vi "datastringtoformat.vi"(0 "object in":refnum<class "interface.lvclass">, 1 "data[0]":string, 5 "error in (no error)":errorcluster) -> (14 "object out":refnum<class "interface.lvclass">, 15 "time stamp":timestamp format="%<%Y/%m/%d %H:%M:%S>T", 19 "error out":errorcluster)   [LabVIEW 2016, in "interface.lvclass"]
uses:
  interface.lvclass
  <vilib>/Utility/miscctls.llb/LVDateTimeRec.ctl
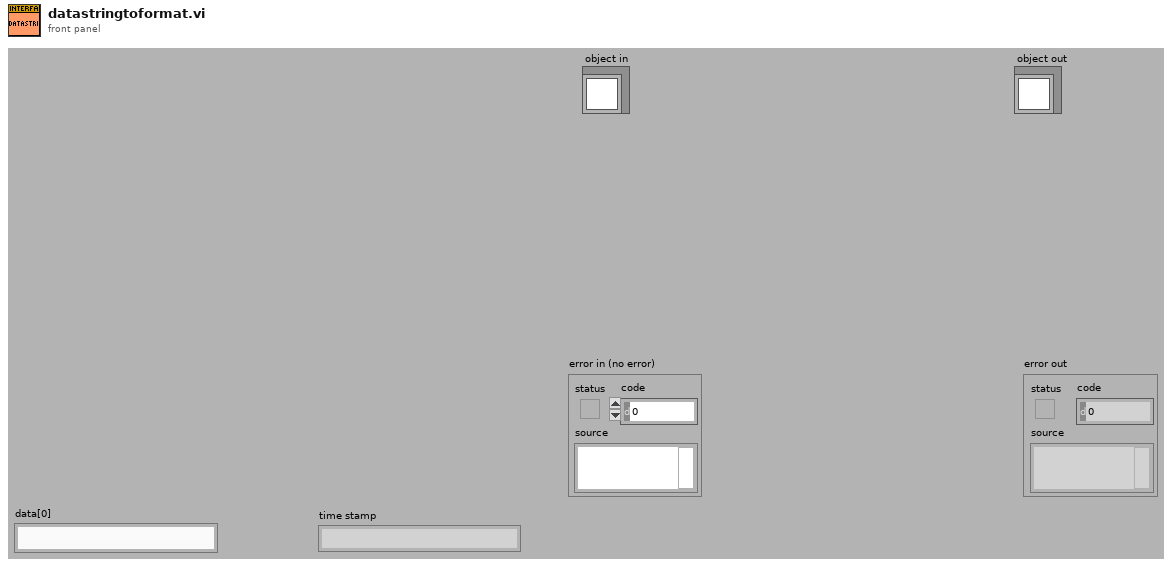
[diagram p1: front panel]
types:
  T1 = typedef "LVDateTimeRec.ctl" = cluster{"fractional second":dbl, "second":i32, "minute":i32, "hour":i32, "day of month":i32, "month":i32, "year":i32, "day of week":i32, "day of year":i32, "DST":i32}
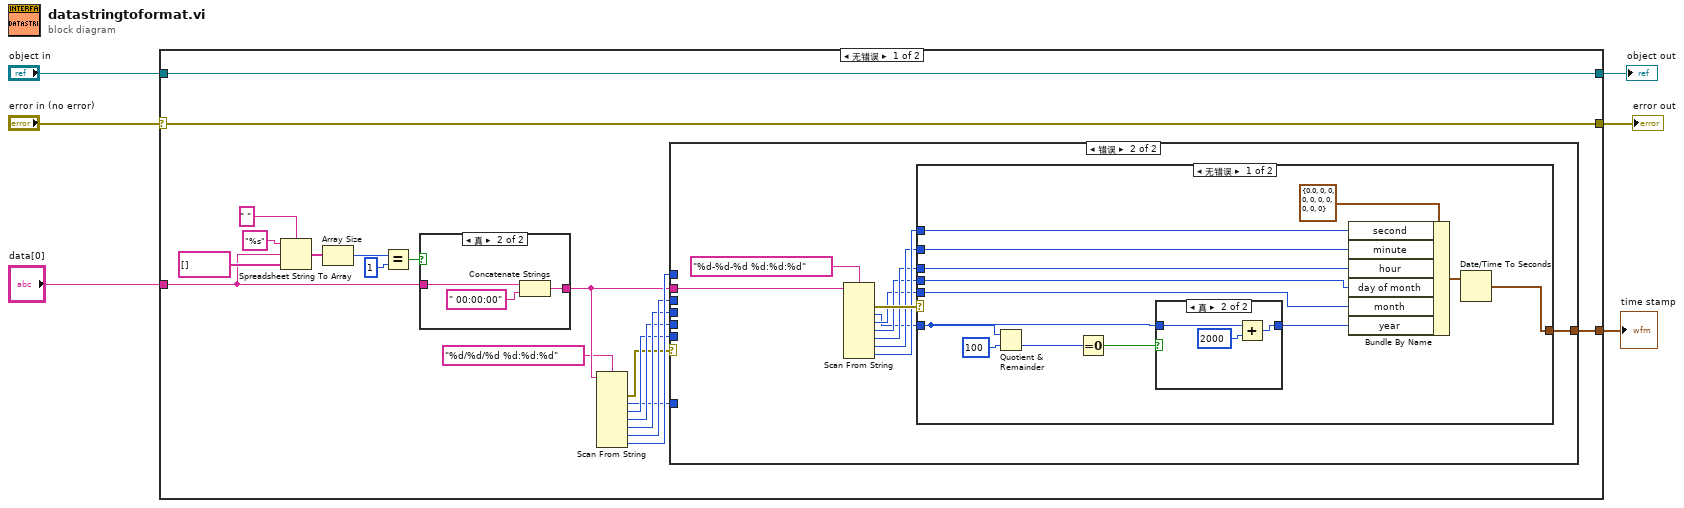
[diagram p0: block diagram]
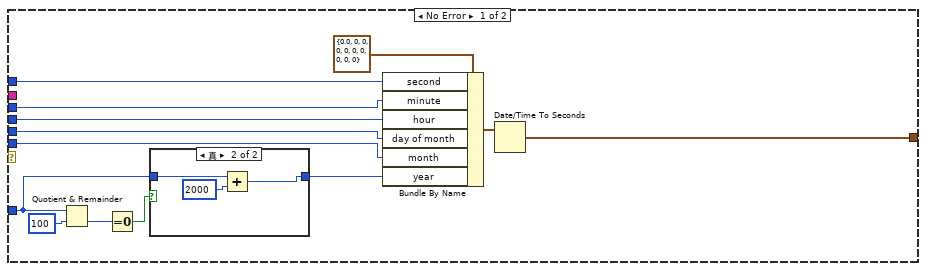
[diagram p3: hidden frame]
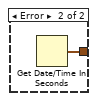
[diagram p6: hidden frame]
diagram:
  n1 = case shown="无错误" "error in (no error)" {
    selector: "error in (no error)" -> [w7 w77]
    tunnel: [w7 w77] -> w5
    tunnel: [w26 w76] -> w3
    tunnel: "object in" -> [w26 w76]
    tunnel: "data[0]" -> [w9 _]
    tunnel: [w8 _] -> w1
    frame No Error {
      n2 = Spreadsheet String To Array(delimiter (Tab)=" " ("分隔符(Tab)"), format string="%s" ("格式字符串"), spreadsheet string=w9, array type (2D Dbl)=string[] []) -> (array=w15:string[])
      n3 = Array Size(array=w15) -> (size(s)=w14:i32)
      n4 = Equal?(x=w14, y=1) -> (x = y?=w12:bool)
      n5 = case shown="真" w12 {
        tunnel: w9 -> [w27 w29]
        tunnel: [w27 w28] -> w11
        frame False {
        }
        frame True {
          n6 = Concatenate Strings(w29, " 00:00:00" ("字符串")) -> (w28:string)
        }
      }
      n7 = Scan From String(format string="%d/%d/%d %d:%d:%d" ("格式字符串"), input string=w11) -> (error out=w19:errorcluster, output 1=w20:i32, output 2=w21:i32, output 3=w22:i32, output 4=w23:i32, output 5=w24:i32, output 6=w25:i32)  [unwired: 8 in, 2 out]
      n8 = case shown="错误" w19 {
        tunnel: w25 -> [w42 _]
        tunnel: w24 -> [w41 _]
        tunnel: w23 -> [w40 _]
        tunnel: w22 -> [w39 _]
        tunnel: w21 -> [w38 _]
        tunnel: w20 -> [w34 _]
        tunnel: [w36 w54] -> w8
        tunnel: w11 -> [_ w57]
        frame No Error {
          n9 = Quotient & Remainder(x=w34, y=100) -> (floor(x/y)=w33:i32)  [unwired: 1 out]
          n10 = Equal To 0?(x=w33) -> (x = 0?=w32:bool)
          n11 = case shown="真" w32 {
            tunnel: w34 -> [w44 w47]
            tunnel: [w44 w45] -> w31
            frame False {
            }
            frame True {
              n12 = Add(x=w47, y=2000) -> (x+y=w45:i32)
            }
          }
          n13 = Bundle By Name(cluster=T1 {"fractional second"=0.0, "second"=0, "minute"=0, "hour"=0, "day of month"=0, "month"=0, "year"=0, "day of week"=0, "day of year"=0, "DST"=0} ("日期时间记录"), "second"=w42, "minute"=w41, "hour"=w40, "day of month"=w39, "month"=w38, "year"=w31) -> (w43:T1)
          n14 = Date/Time To Seconds(2:w43) -> (0:w36:timestamp)  [unwired: 1 in]
        }
        frame Error {
          n15 = Scan From String(format string="%d-%d-%d %d:%d:%d" ("格式字符串"), input string=w57) -> (error out=w55:errorcluster, output 1=w48:i32, output 2=w49:i32, output 3=w50:i32, output 4=w51:i32, output 5=w52:i32, output 6=w53:i32)  [unwired: 8 in, 2 out]
          n16 = case shown="无错误" w55 {
            tunnel: [w64 w75] -> w54
            tunnel: w53 -> [w63 _]
            tunnel: w52 -> [w62 _]
            tunnel: w51 -> [w61 _]
            tunnel: w50 -> [w60 _]
            tunnel: w49 -> [w59 _]
            tunnel: w48 -> [w58 _]
            frame No Error {
              n17 = Quotient & Remainder(x=w58, y=100) -> (floor(x/y)=w67:i32)  [unwired: 1 out]
              n18 = Equal To 0?(x=w67) -> (x = 0?=w66:bool)
              n19 = case shown="真" w66 {
                tunnel: w58 -> [w71 w74]
                tunnel: [w71 w72] -> w65
                frame False {
                }
                frame True {
                  n20 = Add(x=w74, y=2000) -> (x+y=w72:i32)
                }
              }
              n21 = Bundle By Name(cluster=T1 {"fractional second"=0.0, "second"=0, "minute"=0, "hour"=0, "day of month"=0, "month"=0, "year"=0, "day of week"=0, "day of year"=0, "DST"=0} ("日期时间记录"), "second"=w63, "minute"=w62, "hour"=w61, "day of month"=w60, "month"=w59, "year"=w65) -> (w70:T1)
              n22 = Date/Time To Seconds(2:w70) -> (0:w64:timestamp)  [unwired: 1 in]
            }
            frame Error {
              n23 = Get Date/Time In Seconds() -> (seconds since 1Jan1904=w75:timestamp)
            }
          }
        }
      }
    }
    frame Error {
    }
  }
  "error out" <- w5
  "object out" <- w3
  "time stamp" <- w1
